vi "Eagle Scanner Survay.vi"() -> ()   [LabVIEW 2015]
uses:
  <vilib>/FPGAPlugInAG/cRIO-9030/niLvFpga_Open_cRIO-9030.vi
  <vilib>/rvi/interface/common/dynamic/niFpgaDynamicAddResources.vi
  <vilib>/FPGAPlugInAG/Dynamic/niLvFpga_Run_Dynamic.vi
  <vilib>/Utility/error.llb/Error Cluster From Error Code.vi
  <vilib>/rvi/errors/niLvFpgaAdjustHostInterfaceError.vi
  <vilib>/rvi/interface/nirviOpenFPGA/nirviOpenFPGA.xnode
  FPGA Bitfiles/BELKINEAGLEGUI_FPGATarget_EagleFPGAScanner_juOkZGXIgM0.lvbitx
  <vilib>/rvi/interface/nirviMethod/nirviMethod.xnode
  <vilib>/rvi/interface/nirviReadWriteControl/nirviReadWriteControl.xnode
  <vilib>/rvi/interface/Simulation/niFpgaSimulationCallBeginRW.vi
  NiFpgaLv.dll
panel:
  out "spreadsheet string":string
  out "error out 2":errorcluster
  out "error out":errorcluster
  out "Y Read Array":fxp<+/-,20,5>[][](array[numeric])
  out "X Read Array":fxp<+/-,20,5>[][](array[numeric])
  in  "Delay":dbl
  in  "Y Array":fxp<+/-,20,5>[](array[numeric])=[-10.0, -9.0, -8.0, -7.0, -6.0, -5.0, -4.0, -3.0, -2.0, -1.0, 0.0, 1.0, 2.0, 3.0, 4.0, 5.0, 6.0, 7.0, 8.0, 9.0, 10.0]
  in  "X Array":fxp<+/-,20,5>[](array[numeric])=[-10.0, -9.0, -8.0, -7.0, -6.0, -5.0, -4.0, -3.0, -2.0, -1.0, 0.0, 1.0, 2.0, 3.0, 4.0, 5.0, 6.0, 7.0, 8.0, 9.0, 10.0]
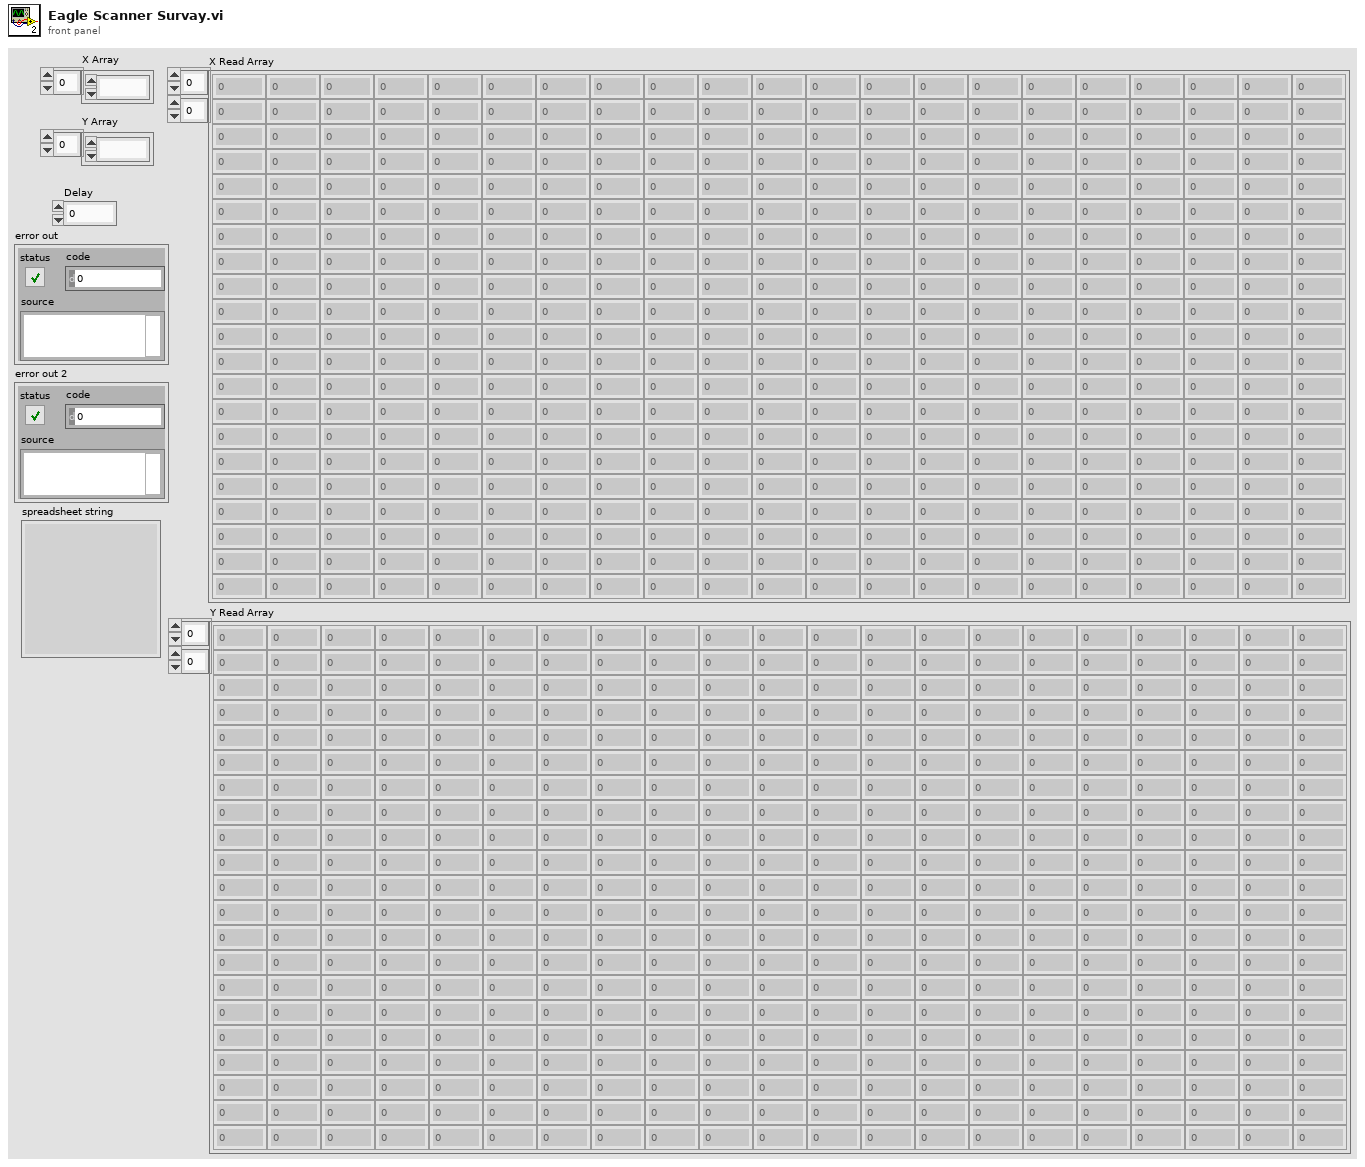
[diagram p1: front panel]
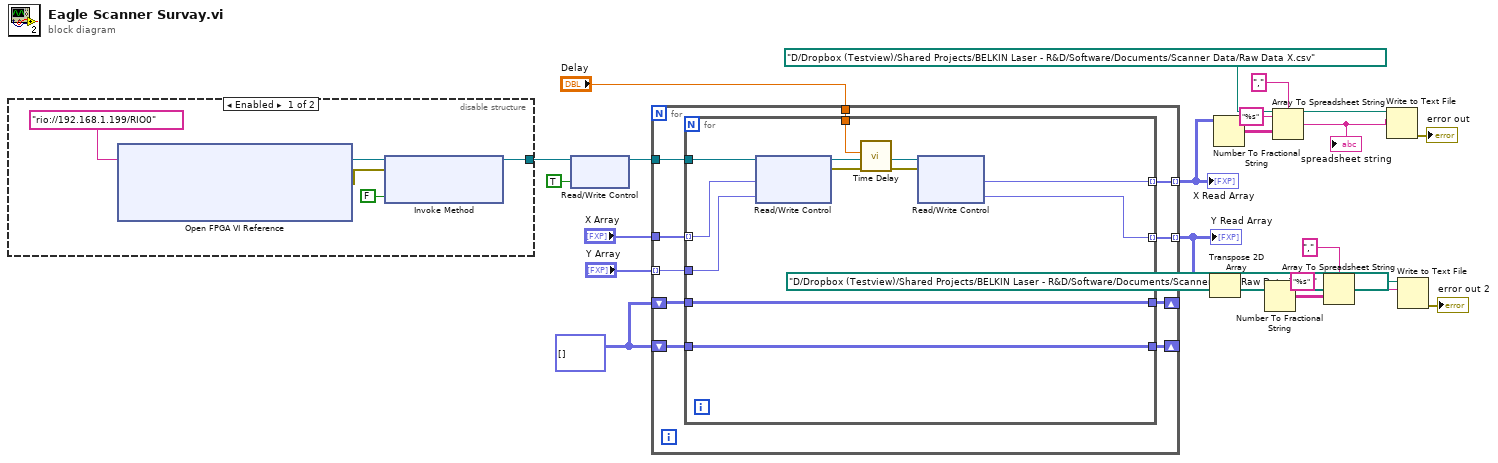
[diagram p0: block diagram]
diagram:
  w16 = fxp<+/-,20,5>[][] [] ("X Read Array")
  n1 = disable-structure shown="Enabled" {
    disable-tunnel: [w23 _] -> w20
    frame Enabled {
      n2 = xnode "Open FPGA VI Reference"("resource name"=tag "rio://192.168.1.199/RIO0") -> ("FPGA VI Reference Out"=w26:refnum<k20>, "error out"=w25:errorcluster)  [unwired: 1 in]
      n3 = xnode "Invoke Method"("FPGA VI Reference In"=w26, "error in"=w25, "Wait Until Done (F)"=FALSE) -> ("FPGA VI Reference Out"=w23:refnum<k20>)  [unwired: 1 out]
    }
    frame Disabled {
    }
  }
  n4 = xnode "Read/Write Control"("FPGA VI Reference In"=w20, "Manual"=TRUE) -> ("FPGA VI Reference Out"=w19:refnum<k20>)  [unwired: 1 in, 1 out]
  n5 = for {
    tunnel: "Y Array" -> [w35] mode=indexing
    tunnel: "X Array" -> [w37]
    tunnel: w19 -> [w36]
    tunnel: "Delay" -> [w34]
    shift-right: [w29] -> _
    shift-left: w16 -> [w33]
    shift-right: [w28] -> _
    shift-left: w16 -> [w30]
    tunnel: [w32] -> w15 mode=indexing
    tunnel: [w31] -> w11 mode=indexing
    n6 = for {
      tunnel: w37 -> [w47] mode=indexing
      tunnel: w36 -> [w48]
      tunnel: w35 -> [w46]
      tunnel: w34 -> [w44]
      tunnel: w33 -> [w39]
      tunnel: [w41] -> w32 mode=indexing
      tunnel: [w40] -> w31 mode=indexing
      tunnel: w30 -> [w38]
      tunnel: [w39] -> w29
      tunnel: [w38] -> w28
      n7 = xnode "Read/Write Control"("FPGA VI Reference In"=w48, "Manual VX"=w47, "Manual VY"=w46) -> ("FPGA VI Reference Out"=w42:refnum<k20>, "error out"=w45:errorcluster)  [unwired: 1 in]
      n8 = call "Time Delay"("error in (no error)"=w45, "Delay Time (s)"=w44) -> ("error out"=w43:errorcluster)  [unwired: 9 in]
      n9 = xnode "Read/Write Control"("FPGA VI Reference In"=w42, "error in"=w43) -> ("X READ 2"=w41:fxp<+/-,20,5>, "Y READ 2"=w40:fxp<+/-,20,5>)  [unwired: 2 out]
    }
  }
  "X Read Array" <- w15
  "Y Read Array" <- w11
  n10 = Transpose 2D Array(2D array=w11) -> (transposed array=w7:fxp<+/-,20,5>[][])
  n11 = Number To Fractional String(number=w15) -> (F-format string=w14:string[][])  [unwired: 3 in]
  n12 = Number To Fractional String(number=w7) -> (F-format string=w8:string[][])  [unwired: 3 in]
  n13 = Array To Spreadsheet String(delimiter (Tab)=",", array=w14, 3:"%s" ("format string")) -> (spreadsheet string=w6:string)
  "spreadsheet string" <- w6
  n14 = Array To Spreadsheet String(delimiter (Tab)=",", array=w8, 3:"%s" ("format string")) -> (spreadsheet string=w4:string)
  n15 = Write to Text File(file (use dialog)=path "D:/Dropbox (Testview)/Shared Projects/BELKIN Laser - R&D/Software/Documents/Scanner Data/Raw Data X.csv", text=w6) -> (error out=→"error out":errorcluster)  [unwired: 2 in, 2 out]
  n16 = Write to Text File(file (use dialog)=path "D:/Dropbox (Testview)/Shared Projects/BELKIN Laser - R&D/Software/Documents/Scanner Data/Raw Data Y.csv", text=w4) -> (error out=→"error out 2":errorcluster)  [unwired: 2 in, 2 out]
